vi "_save_csv_phaseCAL_Ken_Steps.vi"(7 "NoteName":string="SingleCh_", 11 "array in":string[][](array[string])) -> ()   [LabVIEW 2023, in "JIO.lvlib"]
uses:
  <vilib>/Utility/file.llb/Write Delimited Spreadsheet (string).vi
  JIO.lvlib
panel:
  out "FileName":string
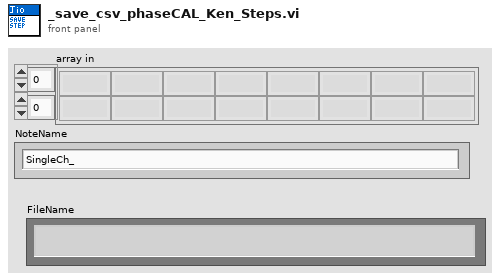
[diagram p1: front panel]
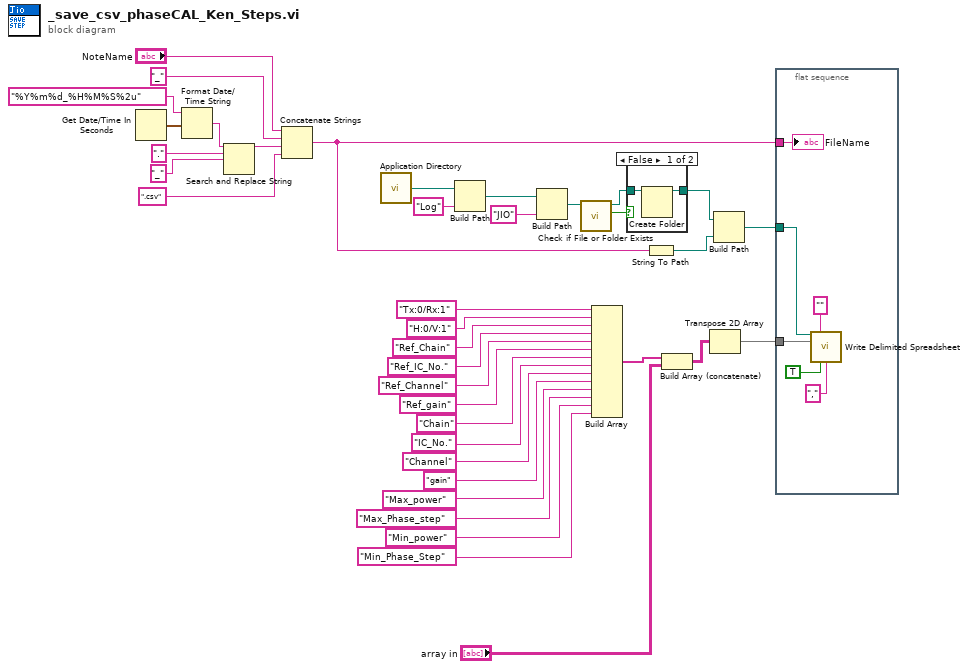
[diagram p0: block diagram]
diagram:
  n1 = Get Date/Time In Seconds() -> (seconds since 1Jan1904=w20:timestamp)
  n2 = Format Date/Time String(time format string (%c)="%Y%m%d_%H%M%S%2u", seconds (now)=w20) -> (date/time string=w18:string)  [unwired: 1 in]
  n3 = Search and Replace String(input string=w18, search string=".", replace string="_") -> (result string=w15:string)  [unwired: 5 in, 3 out]
  n4 = Concatenate Strings("NoteName", "_", w15, ".csv" ("delimiter (\\t)")) -> (w35:string)
  n5 = call <vilib>:"Application Directory.vi"() -> ("Application Directory"=w12:path)
  n6 = Build Path(base path=w12, name or relative path="Log") -> (appended path=w10:path)
  n7 = Build Path(base path=w10, name or relative path="JIO") -> (appended path=w9:path)
  n8 = call <vilib>:"Check if File or Folder Exists.vi"("path"=w9) -> ("file or folder exists?"=w34:bool, "dup path"=w33:path)  [unwired: 8 in, 1 out]
  n9 = Build Array("Tx:0/Rx:1", "H:0/V:1", "Ref_Chain", "Ref_IC_No.", "Ref_Channel", "Ref_gain", "Chain", "IC_No.", "Channel", "gain", "Max_power", "Max_Phase_step", "Min_power", "Min_Phase_Step") -> (w23:string[])
  n10 = case shown="False" w34 {
    tunnel: w33 -> [w40 w41]
    tunnel: [w39 w41] -> w32
    frame False {
      n11 = Create Folder(path (use dialog)=w40) -> (created path=w39:path)  [unwired: 2 in, 2 out]
    }
    frame True {
    }
  }
  n12 = String To Path(string=w35) -> (path=w37:path)
  n13 = Build Array (concatenate)(w23, "array in") -> (w29:string[][])
  n14 = Transpose 2D Array(2D array=w29) -> (transposed array=w31:string[][])
  n15 = Build Path(base path=w32, name or relative path=w37) -> (appended path=w36:path)
  n16 = flat-sequence {
    tunnel: w36 -> [w46]
    tunnel: w35 -> [w44]
    tunnel: w31 -> [w42]
    frame #0 {
      n17 = call-poly <vilib>:"Write Delimited Spreadsheet.vi"("file path (dialog if empty)"=w46, "format (%s)"="" ("format (%.3f)"), "2D data"=w42, "transpose? (no:F)"=TRUE, "delimiter (\\t)"="," ("delimiter (\\t)")) -> ()  [unwired: 9 in, 2 out]
      "FileName" <- w44
    }
  }
